vi "set PG according to private data.vi"(8 "error in (no error)":errorcluster, 11 "Pulse Gen Scan in":refnum<class "Pulse Gen Scan.lvclass">) -> (0 "error out":errorcluster, 3 "Pulse Gen Scan out":refnum<class "Pulse Gen Scan.lvclass">)   [LabVIEW 2009, in "Pulse Gen Scan.lvclass"]
uses:
  Pulse Gen Scan.lvclass
  Pulse Gen Scan.lvclass/Pulse Gen Scan.ctl
  Instruments/Utility Classes/Scannable/Scannable.lvclass
panel:
  out "Outputs on/off":bool[](array[boolean])
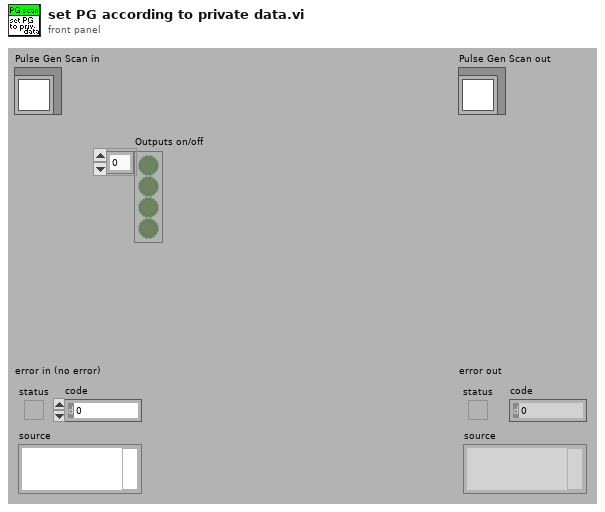
[diagram p1: front panel]
types:
  T1 = enum16{"Channel All ", "Channel 1", "Channel 2", "Channel 3", "Channels Combined"}
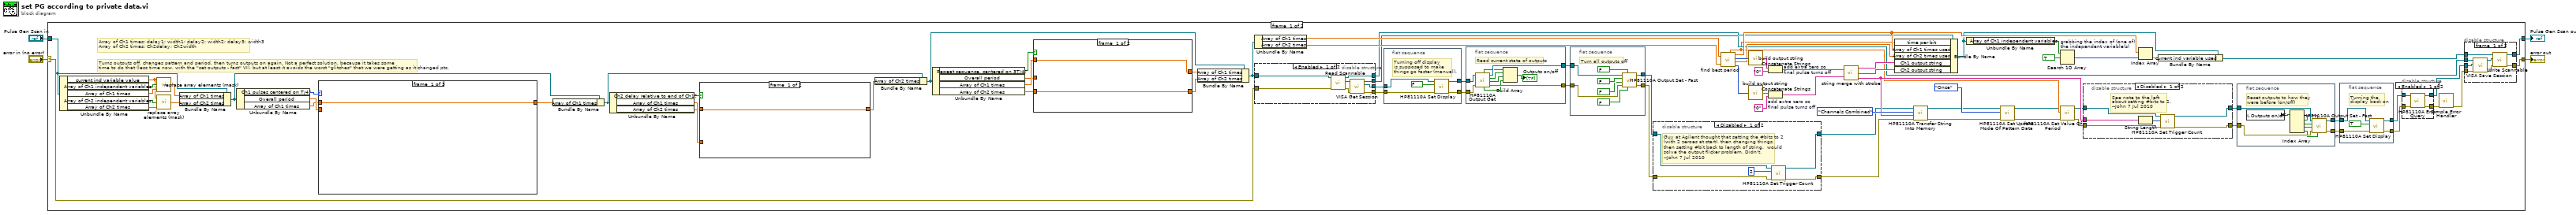
[diagram p0: block diagram]
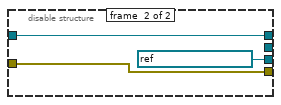
[diagram p3: hidden frame]
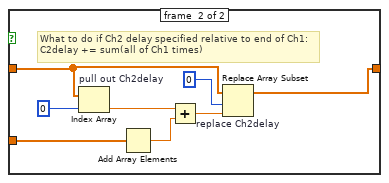
[diagram p7: hidden frame]
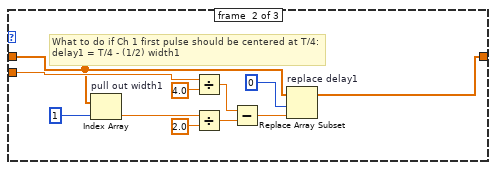
[diagram p8: hidden frame]
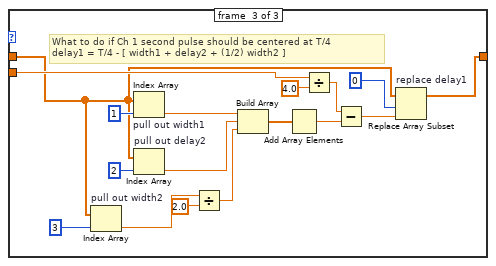
[diagram p9: hidden frame]
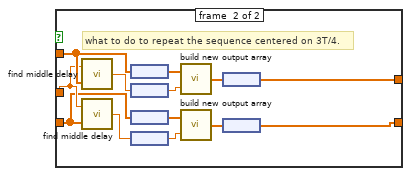
[diagram p10: hidden frame]
diagram:
  n1 = case shown="No Error" "error in (no error)" {
    selector: "error in (no error)" -> [w32 w216]
    tunnel: [w26 w216] -> w3
    tunnel: "Pulse Gen Scan in" -> [w56 w215]
    tunnel: [w24 w215] -> w1
    frame #0 {
      # "Turns outputs off, changes pattern and period, then turns outputs on again. Not a perfect solution, because it takes some \ntime to do that (less time now, with the \"set outputs - fast\" VI), but at least it avoids the worst \"glitches\" that we were getting as it changed pts."
      # "Array of Ch1 times: delay1; width1; delay2; width2; delay3; width3\nArray of Ch2 times: Ch2delay; Ch2width"
      n2 = Unbundle By Name(w56) -> ("current ind variable value"=w55:dbl[unit], "Array of Ch1 independent variables"=w61:bool[], "Array of Ch1 times"=w60:dbl[unit][], "Array of Ch2 independent variables"=w54:bool[], "Array of Ch2 times"=w53:dbl[unit][])
      n3 = call "replace array elements (mask).vi"("input array of numbers"=w60, "array of booleans (mask)"=w61, "value"=w55) -> ("output array"=w57:dbl[unit][])
      n4 = call "replace array elements (mask).vi"("input array of numbers"=w53, "array of booleans (mask)"=w54, "value"=w55) -> ("output array"=w52:dbl[unit][])
      n5 = Bundle By Name(cluster=w56, "Array of Ch1 times"=w57, "Array of Ch2 times"=w52) -> (w50:refnum<class "Pulse Gen Scan.lvclass">)
      n6 = Unbundle By Name(w50) -> ("Ch1 pulses centered on T/4?"=w79:enum32{"none", "first", "second"}, "Overall period"=w59:dbl[unit], "Array of Ch1 times"=w58:dbl[unit][])
      n7 = case shown="\"second\"" w79 {
        tunnel: w58 -> [w171 w173 w185]
        tunnel: [w171 w175 w191] -> w51
        tunnel: w59 -> [_ w176 w192]
        frame #0 {
        }
        frame #1 {
          # "What to do if Ch 1 first pulse should be centered at T/4:\ndelay1 = T/4 - (1/2) width1"
          n8 = Index Array "pull out width1"(array=w173, index=1) -> (element=w172:dbl[unit])
          n9 = Divide(x=w176, y=4.0) -> (x/y=w181:dbl[unit])
          n10 = Divide(x=w172, y=2.0) -> (x/y=w179:dbl[unit])
          n11 = Subtract(x=w181, y=w179) -> (x-y=w177:dbl[unit])
          n12 = Replace Array Subset "replace delay1"(array=w173, new element=w177, index=0) -> (w175:dbl[unit][])
        }
        frame #2 {
          # "What to do if Ch 1 second pulse should be centered at T/4\ndelay1 = T/4 - [ width1 + delay2 + (1/2) width2 ]"
          n13 = Index Array "pull out width2"(array=w185, index=3) -> (element=w184:dbl[unit])
          n14 = Index Array "pull out width1"(array=w185, index=1) -> (element=w189:dbl[unit])
          n15 = Index Array "pull out delay2"(array=w185, index=2) -> (element=w187:dbl[unit])
          n16 = Divide(x=w184, y=2.0) -> (x/y=w194:dbl[unit])
          n17 = Build Array(w189, w187, w194) -> (w196:dbl[unit][])
          n18 = Add Array Elements(numeric array=w196) -> (sum=w195:dbl[unit])
          n19 = Divide(x=w192, y=4.0) -> (x/y=w198:dbl[unit])
          n20 = Subtract(x=w198, y=w195) -> (x-y=w183:dbl[unit])
          n21 = Replace Array Subset "replace delay1"(array=w185, new element=w183, index=0) -> (w191:dbl[unit][])
        }
      }
      n22 = Bundle By Name(cluster=w50, "Array of Ch1 times"=w51) -> (w33:refnum<class "Pulse Gen Scan.lvclass">)
      n23 = Unbundle By Name(w33) -> ("Ch2 delay relative to end of Ch1?"=w45:bool, "Array of Ch1 times"=w49:dbl[unit][], "Array of Ch2 times"=w44:dbl[unit][])
      n24 = case shown="True" w45 {
        tunnel: [w162 w165] -> w48
        tunnel: w44 -> [w162 w163]
        tunnel: w49 -> [_ w169]
        frame #0 {
        }
        frame #1 {
          # "What to do if Ch2 delay specified relative to end of Ch1:\nC2delay += sum(all of Ch1 times)"
          n25 = Index Array "pull out Ch2delay"(array=w163, index=0) -> (element=w164:dbl[unit])
          n26 = Add Array Elements(numeric array=w169) -> (sum=w170:dbl[unit])
          n27 = Add(x=w164, y=w170) -> (x+y=w166:dbl[unit])
          n28 = Replace Array Subset "replace Ch2delay"(array=w163, new element=w166, index=0) -> (w165:dbl[unit][])
        }
      }
      n29 = Bundle By Name(cluster=w33, "Array of Ch2 times"=w48) -> (w41:refnum<class "Pulse Gen Scan.lvclass">)
      n30 = Unbundle By Name(w41) -> ("Repeat sequence, centered on 3T/4?"=w42:bool, "Overall period"=w43:dbl[unit], "Array of Ch1 times"=w46:dbl[unit][], "Array of Ch2 times"=w47:dbl[unit][])
      n31 = case shown="True" w42 {
        tunnel: w46 -> [w201 w208]
        tunnel: [w201 w211] -> w39
        tunnel: w47 -> [w200 w203]
        tunnel: [w200 w209] -> w37
        tunnel: w43 -> [_ w206]
        frame #0 {
        }
        frame #1 {
          # "what to do to repeat the sequence centered on 3T/4."
          n32 = call "find middle delay.vi"("array of times"=w208, "Expected overall period"=w206) -> ("middle delay"=w207:dbl[unit])
          n33 = call "find middle delay.vi"("array of times"=w203, "Expected overall period"=w206) -> ("middle delay"=w205:dbl[unit])
          n34 = node(w208) -> (w214:dbl[])
          n35 = node(w207) -> (w213:dbl)
          n36 = node(w203) -> (w202:dbl[])
          n37 = node(w205) -> (w204:dbl)
          n38 = call "build new output array.vi"("number to insert"=w213, "input array"=w214) -> ("output array"=w212:dbl[])
          n39 = call "build new output array.vi"("number to insert"=w204, "input array"=w202) -> ("output array"=w210:dbl[])
          n40 = node(w212) -> (w211:dbl[unit][])
          n41 = node(w210) -> (w209:dbl[unit][])
        }
      }
      n42 = Bundle By Name(cluster=w41, "Array of Ch1 times"=w39, "Array of Ch2 times"=w37) -> (w30:refnum<class "Pulse Gen Scan.lvclass">)
      n43 = Unbundle By Name(w30) -> ("Array of Ch1 times"=w40:dbl[unit][], "Array of Ch2 times"=w38:dbl[unit][])
      n44 = disable-structure shown="Enabled" {
        disable-tunnel: w32 -> [w100 w104]
        disable-tunnel: [w99 w105] -> w31
        disable-tunnel: w30 -> [w98 w105]
        disable-tunnel: [w97 _] -> w28
        disable-tunnel: [w96 refnum<visa-resource-name> "GPIB0::10::INSTR" ("VISA Resource Name")] -> w23
        disable-tunnel: [w95 w104] -> w21
        frame #0 {
          n45 = call-dynamic "Read Scannable.vi"("error in (no error)"=w100, "Scanner.lvclass in"=w98) -> ("error out"=w101:errorcluster, "Scannable.lvclass"=w102:refnum<class "Scannable.lvclass">, "Scanner.lvclass out"=w99:refnum<class "Pulse Gen Scan.lvclass">)  [unwired: 7 out]
          n46 = call-dynamic "VISA Get Session.vi"("error in (no error)"=w101, "Instrument.lvclass in"=w102) -> ("error out"=w95:errorcluster, "VISA Resource Name"=w96:refnum<visa-resource-name>, "Instrument.lvclass out"=w97:refnum<class "Scannable.lvclass">)  [unwired: 7 out]
        }
        frame #1 {
        }
      }
      n47 = flat-sequence {
        tunnel: w23 -> [w123]
        tunnel: [w122] -> w22
        tunnel: w21 -> [w121]
        tunnel: [w120] -> w20
        frame #0 {
          # "Turning off display\nis supposed to make \nthings go faster (manual)."
          n48 = call "HP81110A Set Display.vi"("error in (no error)"=w121, "Display (F:Off)"=FALSE, "VISA session"=w123) -> ("error out"=w120:errorcluster, "dup VISA session"=w122:refnum<visa-resource-name>)  [unwired: 7 out]
        }
      }
      n49 = flat-sequence {
        tunnel: [w141] -> w69
        tunnel: [w140] -> w68
        tunnel: w20 -> [w139]
        tunnel: w22 -> [w138]
        frame #0 {
          # "Read current state of outputs"
          n50 = call "HP81110A Output Get.vi"("error in (no error)"=w139, "VISA session"=w138) -> ("error out"=w140:errorcluster, "output2OUT"=w135:bool, "notoutput1OUT"=w136:bool, "dup VISA session"=w141:refnum<visa-resource-name>, "notoutput2OUT"=w134:bool, "output1OUT"=w137:bool)  [unwired: 4 out]
          n51 = Build Array(w137, w136, w135, w134) -> (→"Outputs on/off":bool[])
        }
      }
      n52 = flat-sequence {
        tunnel: w69 -> [w132]
        tunnel: w68 -> [w131]
        tunnel: [w130] -> w19
        tunnel: [w129] -> w18
        frame #0 {
          # "Turn all outputs off"
          n53 = call "HP81110A Output Set - Fast.vi"("notoutput2"=FALSE, "output1"=FALSE, "error in (no error)"=w131, "output2"=FALSE, "notoutput1"=FALSE, "VISA session"=w132) -> ("error out"=w129:errorcluster, "dup VISA session"=w130:refnum<visa-resource-name>)  [unwired: 4 out]
        }
      }
      n54 = disable-structure shown="Disabled" {
        disable-tunnel: w19 -> [w153 w156]
        disable-tunnel: w18 -> [w152 w155]
        disable-tunnel: [w151 w155] -> w11
        disable-tunnel: [w150 w156] -> w12
        frame #0 {
          # "Guy at Agilent thought that setting the #bits to 2 \n(with 2 zeroes at start), then changing things, \nthen setting #bit back to length of string,  would \nsolve the output flicker problem. Didn't.\n--John 7 Jul 2010"
          n55 = call "HP81110A Set Trigger Count.vi"("error in (no error)"=w152, "Trigger Count"=2, "VISA session"=w153) -> ("error out"=w151:errorcluster, "dup VISA session"=w150:refnum<visa-resource-name>)  [unwired: 7 out]
        }
        frame #1 {
        }
      }
      n56 = call "find best period.vi"("Array of Ch2 desired times"=w38, "Array of Ch1 desired times"=w40) -> ("Array of Ch2 \"period-units\""=w83:i32[], "Array of Ch2 actual times"=w77:dbl[unit][], "Array of Ch1 \"period-units\""=w84:i32[], "Array of Ch1 actual times"=w78:dbl[unit][], "best period"=w17:dbl[unit])
      n57 = call "build output string.vi"("Array of \"period-units\""=w84) -> ("output string"=w73:string)
      n58 = call "build output string.vi"("Array of \"period-units\""=w83) -> ("output string"=w72:string)
      n59 = Concatenate Strings "add extra zero so \nfinal pulse turns off"(w73, "0" ("string")) -> (w67:string)
      n60 = Concatenate Strings "add extra zero so \nfinal pulse turns off"(w72, "0" ("string")) -> (w66:string)
      n61 = call "string merge with strobe.vi"("Ch1 String"=w67, "Ch2 String"=w66) -> ("Ch1 Output String"=w35:string, "Ch2 Output String"=w34:string, "Merged Output String"=w62:string)
      n62 = Bundle By Name(cluster=w31, "time per bit"=w17, "Array of Ch1 times used"=w78, "Array of Ch2 times used"=w77, "Ch1 output string"=w35, "Ch2 output string"=w34) -> (w36:refnum<class "Pulse Gen Scan.lvclass">)
      n63 = call "HP81110A Transfer String Into Memory.vi"("error in (no error)"=w11, "String"=w62, "Channel (1:Channel 1)"=T1."Channels Combined", "VISA session"=w12) -> ("error out"=w63:errorcluster, "dup VISA session"=w64:refnum<visa-resource-name>)  [unwired: 6 out]
      n64 = Unbundle By Name(w36) -> ("Array of Ch1 independent variables"=w81:bool[])
      n65 = call "HP81110A Set Update Mode Of Pattern Data.vi"("error in (no error)"=w63, "Pattern Update Mode (1:Continuous)"=enum16{"Off", "Continuous", "Once"}."Once", "VISA session"=w64) -> ("error out"=w14:errorcluster, "dup VISA session"=w16:refnum<visa-resource-name>)  [unwired: 7 out]
      n66 = Search 1D Array "grabbing the index of (one of) \nthe independent variable(s)"(1D array=w81, element=TRUE) -> (index of element=w80:i32)  [unwired: 1 out]
      n67 = call "HP81110A Set Value Of Period.vi"("error in (no error)"=w14, "Period Value"=w17, "VISA session"=w16) -> ("error out"=w13:errorcluster, "dup VISA session"=w15:refnum<visa-resource-name>)  [unwired: 7 out]
      n68 = disable-structure shown="Disabled" {
        disable-tunnel: [w146 w149] -> w6
        disable-tunnel: [w145 w148] -> w5
        disable-tunnel: w15 -> [w144 w149]
        disable-tunnel: w13 -> [w143 w148]
        disable-tunnel: w62 -> [w142 _]
        frame #0 {
          # "See note to the left \nabout setting #bits to 2.\n--John 7 Jul 2010"
          n69 = String Length(string=w142) -> (length=w147:i32)
          n70 = call "HP81110A Set Trigger Count.vi"("error in (no error)"=w143, "Trigger Count"=w147, "VISA session"=w144) -> ("error out"=w145:errorcluster, "dup VISA session"=w146:refnum<visa-resource-name>)  [unwired: 7 out]
        }
        frame #1 {
        }
      }
      n71 = Index Array(array=w78, index=w80) -> (element=w76:dbl[unit])
      n72 = Bundle By Name(cluster=w36, "current ind variable used"=w76) -> (w25:refnum<class "Pulse Gen Scan.lvclass">)
      n73 = flat-sequence {
        tunnel: [w119] -> w9
        tunnel: [w118] -> w7
        tunnel: w6 -> [w117]
        tunnel: w5 -> [w116]
        frame #0 {
          # "Reset outputs to how they \nwere before (on/off)"
          n74 = local read "Outputs on/off"() -> (w115:bool[])
          n75 = Index Array(array=w115) -> (element #1=w114:bool, element #2=w113:bool, element #3=w112:bool, element #4=w111:bool)  [unwired: 4 in]
          n76 = call "HP81110A Output Set - Fast.vi"("notoutput2"=w111, "output1"=w114, "error in (no error)"=w116, "output2"=w112, "notoutput1"=w113, "VISA session"=w117) -> ("error out"=w118:errorcluster, "dup VISA session"=w119:refnum<visa-resource-name>)  [unwired: 4 out]
        }
      }
      n77 = flat-sequence {
        tunnel: [w109] -> w10
        tunnel: w9 -> [w108]
        tunnel: [w107] -> w8
        tunnel: w7 -> [w106]
        frame #0 {
          # "Turning the \ndisplay back on"
          n78 = call "HP81110A Set Display.vi"("error in (no error)"=w106, "Display (F:Off)"=TRUE, "VISA session"=w108) -> ("error out"=w107:errorcluster, "dup VISA session"=w109:refnum<visa-resource-name>)  [unwired: 7 out]
        }
      }
      n79 = disable-structure shown="Enabled" {
        disable-tunnel: [w160 w161] -> w70
        disable-tunnel: w10 -> [w159 _]
        disable-tunnel: w8 -> [w158 w161]
        disable-tunnel: [w157 _] -> w29
        frame #0 {
          n80 = call "HP81110A Error Query.vi"("VISA session"=w159, "error in (no error)"=w158) -> ("dup VISA session"=w157:refnum<visa-resource-name>, "error out"=w160:errorcluster)  [unwired: 12 out]
        }
        frame #1 {
        }
      }
      n81 = call <vilib>:"Simple Error Handler.vi"("error in (no error)"=w70) -> ("error out"=w27:errorcluster)  [unwired: 1 in, 7 out]
      n82 = disable-structure shown="Enabled" {
        disable-tunnel: w29 -> [w92 _]
        disable-tunnel: w28 -> [w91 _]
        disable-tunnel: w27 -> [w89 w93]
        disable-tunnel: [w88 w93] -> w26
        disable-tunnel: w25 -> [w87 w94]
        disable-tunnel: [w86 w94] -> w24
        frame #0 {
          n83 = call-dynamic "VISA Save Session.vi"("error in (no error)"=w89, "VISA Resource Name"=w92, "Instrument.lvclass in"=w91) -> ("error out"=w90:errorcluster, "Instrument.lvclass out"=w85:refnum<class "Scannable.lvclass">)  [unwired: 7 out]
          n84 = call-dynamic "Write Scannable.vi"("error in (no error)"=w90, "Scannable.lvclass"=w85, "Scanner.lvclass in"=w87) -> ("error out"=w88:errorcluster, "Scanner.lvclass out"=w86:refnum<class "Pulse Gen Scan.lvclass">)  [unwired: 7 out]
        }
        frame #1 {
        }
      }
    }
    frame #1 {
    }
  }
  "error out" <- w3
  "Pulse Gen Scan out" <- w1
